vi "_miopen.vi"(2 "错误输入（无错误）":errorcluster, 3 "数据输入":string, 4 "port":u16=1234, 5 "ip":string="192.168.1.44") -> (0 "错误输出":errorcluster, 1 "连接ID":refnum<k5>)   [LabVIEW 2017]
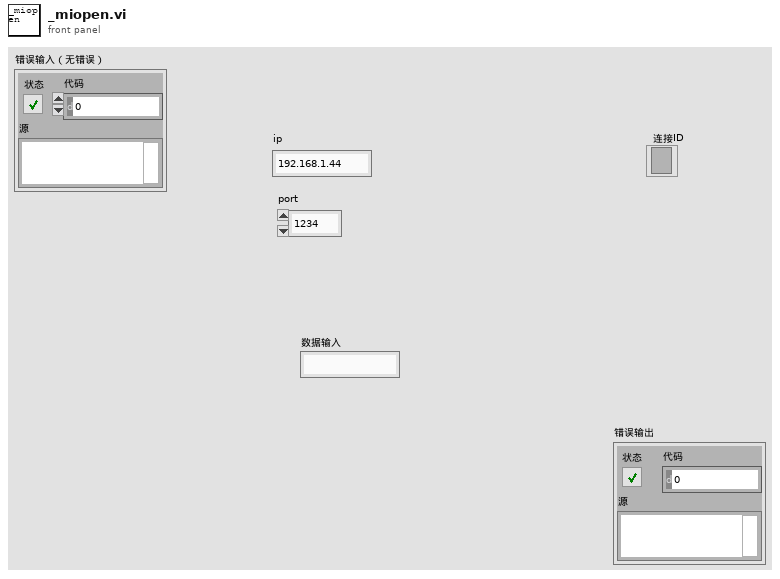
[diagram p1: front panel]
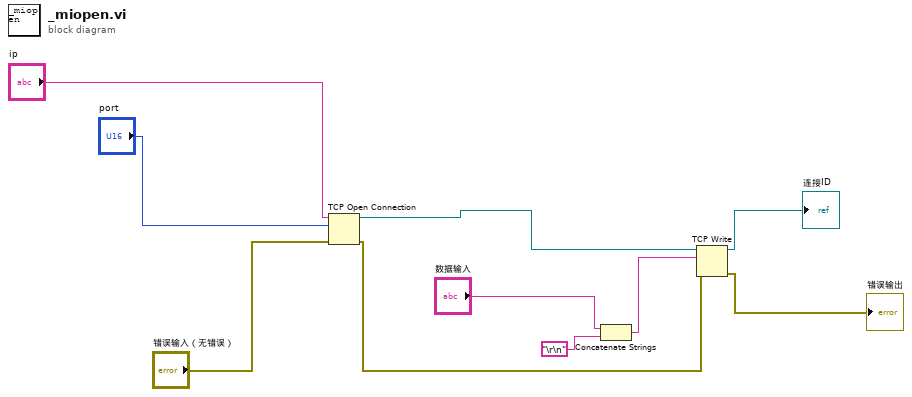
[diagram p0: block diagram]
diagram:
  n1 = TCP Open Connection(address="ip", remote port or service name="port", error in (no error)="错误输入（无错误）") -> (connection ID=w8:refnum<k5>, error out=w7:errorcluster)  [unwired: 2 in]
  n2 = Concatenate Strings("数据输入", "\r\n") -> (w3:string)
  n3 = TCP Write(connection ID=w8, data in=w3, error in (no error)=w7) -> (connection ID out=→"连接ID":refnum<k5>, error out=→"错误输出":errorcluster)  [unwired: 1 in, 1 out]
